vi "Do Core.vi"(8 "error in (no error)":errorcluster, 9 "Actor in":refnum<class "Actor.lvclass">, 11 "Reply Message":refnum<class "Reply Msg.lvclass">) -> (0 "error out":errorcluster, 1 "Actor out":refnum<class "Actor.lvclass">, 2 "Reply":variant)   [LabVIEW 2020, in "AF Specialty Messages.lvlib" / "Reply Msg.lvclass"]
doc: "<p>(<strong>Filename</strong>: <span class=\"dnl\">Actor Framework.lvlib:Reply Msg.lvclass:Do Core.vi</span>)</p>\n<p>Defines what an actor does when it receives <strong>Reply Message</strong>. This method also defines the <strong>Reply</strong> that is returned to the actor that sent <strong>Reply Message</strong>.</p>\n<p>By default, this method does nothing, and <strong>Reply</strong> is the ancestor Message class. A child class must override this method to define behavior and specify a child of the Message class to return in the <strong>Reply</strong> output.</p>"
uses:
  Reply Msg.lvclass
  Actor/Actor.lvclass
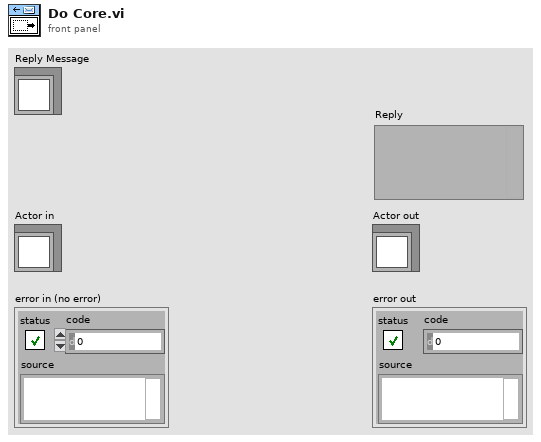
[diagram p1: front panel]
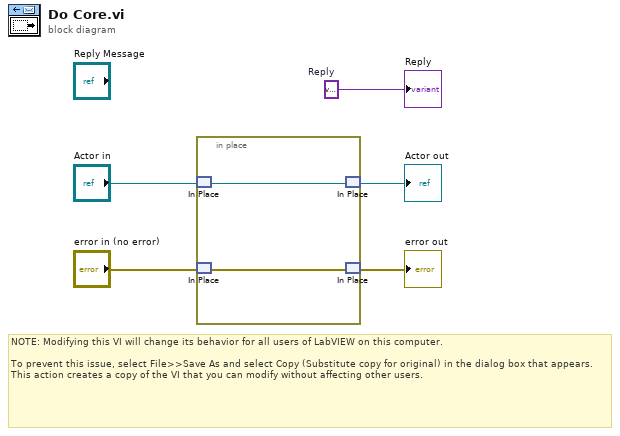
[diagram p0: block diagram]
diagram:
  w1 = variant  # Reply
  # "NOTE: Modifying this VI will change its behavior for all users of LabVIEW on this computer.\n\nTo prevent this issue, select File>>Save As and select Copy (Substitute copy for original) in the dialog box that appears. This action creates a copy of the VI that you can modify without affecting other users."
  n1 = in-place {
    n2 = in-place-match #1("Actor in") -> (w6:refnum<class "Actor.lvclass">)
    n3 = in-place-match #2("error in (no error)") -> (w7:errorcluster)
    n4 = in-place-match #1(w6) -> (→"Actor out":refnum<class "Actor.lvclass">)
    n5 = in-place-match #2(w7) -> (→"error out":errorcluster)
  }
  "Reply" <- w1
